vi "Image Processing.vi"(0 "Image In":T1, 7 "error in":errorcluster) -> (20 "Image Out":T1, 21 "Matches (Pattern Matching 1)":T2(array[cluster]) {"Bounding Box"."y" format="%.2f"; "Bounding Box"."x" format="%.2f"; "Position"."y" format="%.2f"; "Position"."x" format="%.2f"; "Score" format="%.2f"; "Scale" format="%.2f"; "Angle" format="%.2f"}, 27 "error out":errorcluster)   [LabVIEW 2018]
uses:
  <vilib>/vision/Image Controls.llb/IMAQ Image.ctl
  <vilib>/vision/Pattern Matching.llb/IMAQ Pattern Match Advanced Options.ctl
  <vilib>/vision/NI_Vision_Development_Module.lvlib
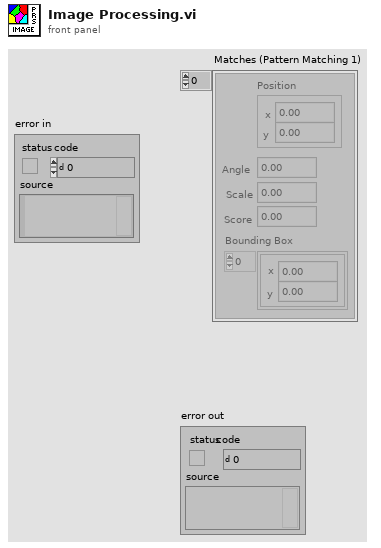
[diagram p1: front panel]
types:
  T1 = typedef "IMAQ Image.ctl" = refnum<image>
  T2 = cluster{"Position":cluster{"x":sgl, "y":sgl}, "Angle":sgl, "Scale":sgl, "Score":sgl, "Bounding Box":cluster{"x":sgl, "y":sgl}[]}[]
  T3 = typedef "IMAQ Pattern Match Advanced Options.ctl" = u16
  T4 = cluster{"Number of Matches Requested":i32, "Minimum Match Score":sgl, "Angle Ranges":cluster{"Start Angle":sgl, "End Angle":sgl}[]}
  T5 = cluster{"Global Rectangle":i32[], "Contours":cluster{"ID":enum32{"External", "Internal"}, "Type":u32, "Coordinates":i32[]}[]}
  T6 = cluster{"Global Rectangle":i32[], "Contours":cluster{"ID":enum32{"External", "Internal"}, "Type":u32, "Coordinates":i32[]}[]}[]
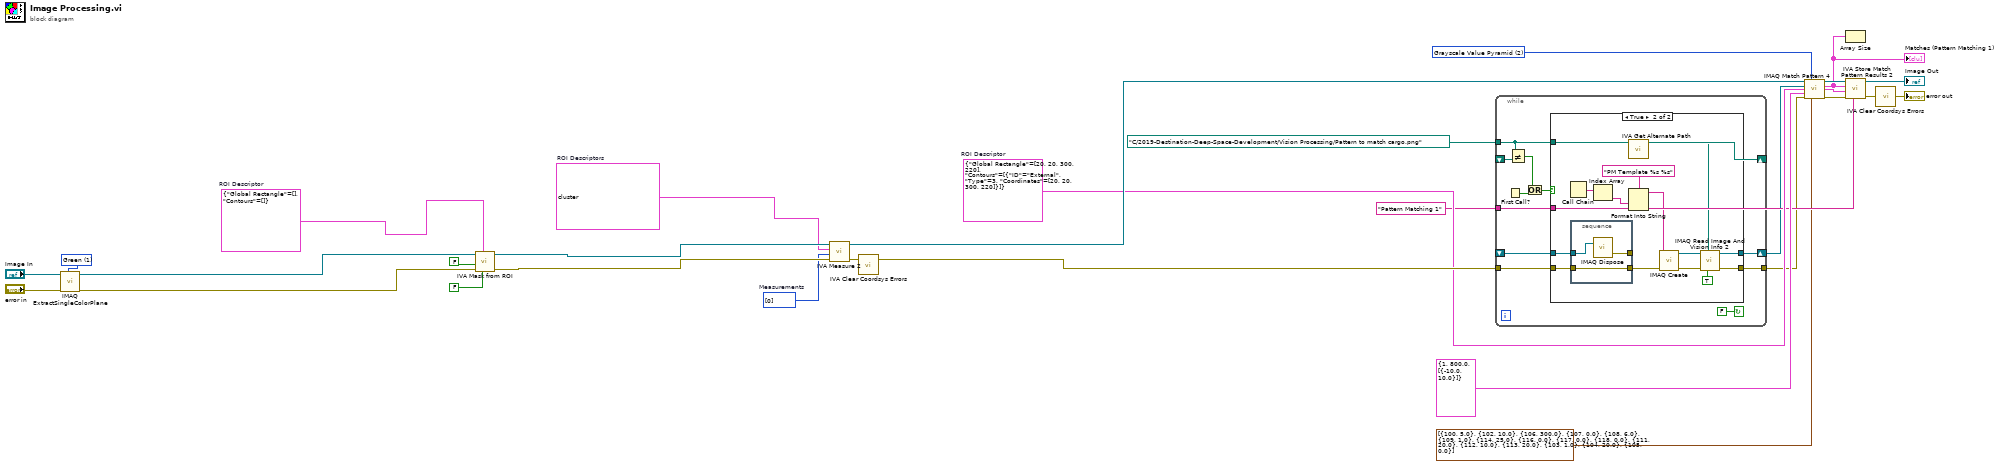
[diagram p0: block diagram]
diagram:
  w11 = 2 items=["All", "Low Discrepancy Sampling", "Grayscale Value Pyramid", "Gradients Pyramid"] ("Algorithm")
  w8 = "Pattern Matching 1" ("Step Name")
  w10 = T5 {"Global Rectangle"=[20, 20, 300, 220], "Contours"=[{"ID"=enum."External", "Type"=3, "Coordinates"=[20, 20, 300, 220]}]}  # ROI Descriptor
  w19 = i32[] [0]  # Measurements
  w20 = T6 [{"Global Rectangle"=[159, 103, 160, 104], "Contours"=[{"ID"=enum."External", "Type"=1, "Coordinates"=[159, 103]}]}]  # ROI Descriptors
  w26 = T5 {"Global Rectangle"=[], "Contours"=[]}  # ROI Descriptor
  w30 = 1 items=["Red", "Green", "Blue", "Hue", "Saturation", "Luminance", "Value", "Intensity"] ("Color Plane")
  n1 = call "IMAQ ExtractSingleColorPlane"("Color Plane"=w30, "error in (no error)"="error in", "Image Src"="Image In") -> ("error out"=w27:errorcluster, "Image Dst Out"=w24:T1)  [unwired: 1 in, 6 out]
  n2 = call <vilib>:"IVA Mask from ROI.vi"("Shrink"=FALSE, "ROI Descriptor"=w26, "error in (no error)"=w27, "Out / In"=FALSE, "Image Src"=w24) -> ("error out"=w22:errorcluster, "Image Out"=w21:T1)  [unwired: 5 out]
  n3 = call <vilib>:"IVA Measure 2.vi"("error in (no error)"=w22, "Measurements"=w19, "ROI Descriptors"=w20, "Image In"=w21) -> ("error out"=w18:errorcluster, "Image Out"=w15:T1)  [unwired: 1 in, 5 out]
  n4 = call <vilib>:"IVA Clear Coordsys Errors.vi"("error in (no error)"=w18) -> ("error out"=w17:errorcluster)  [unwired: 10 in]
  n5 = while {
    shift-right: [w41] -> w5
    shift-left: _ -> [w40]
    tunnel: [w38] -> w4
    tunnel: w17 -> [w37]
    tunnel: path "C:/2019-Destination-Deep-Space-Development/Vision Processing/Pattern to match cargo.png" ("Template File Path") -> [w34]
    tunnel: w8 -> [w36]
    shift-right: [w34] -> _
    shift-left: _ -> [w35]
    stop <- FALSE continue-if-true
    n6 = First Call?() -> (First Call?: T/F=w33:bool)
    n7 = Not Equal?(x=w34, y=w35) -> (x != y?=w32:bool)
    n8 = Or(x=w32, y=w33) -> (x .or. y?=w31:bool)
    n9 = case shown="True" w31 {
      tunnel: [w43 w48] -> w41
      tunnel: w40 -> [w43 w52]
      tunnel: [w42 w49] -> w38
      tunnel: w37 -> [w42 w51]
      tunnel: w34 -> [_ w53]
      tunnel: w36 -> [_ w54]
      frame False {
      }
      frame True {
        n10 = Call Chain() -> (call chain=w56:string[])
        n11 = stacked-sequence {
          tunnel: w52 -> [w61]
          tunnel: w51 -> [w60]
          tunnel: [w60] -> w45
          tunnel: [w59] -> _
          frame #0 {
            n12 = call "IMAQ Dispose"("Image"=w61) -> ("error out"=w59:errorcluster)  [unwired: 2 in, 3 out]
          }
        }
        n13 = Index Array(array=w56) -> (element=w55:string)  [unwired: 1 in]
        n14 = call <vilib>:"IVA Get Alternate Path.vi"("Path In"=w53) -> ("Path Out"=w50:path)  [unwired: 10 out]
        n15 = Format Into String(format string="PM Template %s %s" ("Image Name"), w55, w54) -> (resulting string=w58:string)  [unwired: 2 in, 1 out]
        n16 = call "IMAQ Create"("Image Name"=w58, "error in (no error)"=w45) -> ("New Image"=w47:T1, "error out"=w46:errorcluster)  [unwired: 2 in, 1 out]
        n17 = call "IMAQ Read Image And Vision Info 2"("Use File Path Image Type"=TRUE, "File Path"=w50, "error in (no error)"=w46, "Image"=w47) -> ("error out"=w49:errorcluster, "Image Out"=w48:T1)  [unwired: 5 in, 1 out]
      }
    }
  }
  n18 = call "IMAQ Match Pattern 4"("Image"=w15, "Algorithm"=w11, "Template Image"=w5, "ROI Descriptor"=w10, "Parameters"=T4 {"Number of Matches Requested"=1, "Minimum Match Score"=800.0, "Angle Ranges"=[{"Start Angle"=-10.0, "End Angle"=10.0}]}, "error in (no error)"=w4, "Advanced Options"=cluster{"Item":T3, "Value":dbl}[] [{"Item"=100, "Value"=5.0}, {"Item"=102, "Value"=10.0}, {"Item"=106, "Value"=300.0}, {"Item"=107, "Value"=0.0}, {"Item"=108, "Value"=6.0}, {"Item"=109, "Value"=1.0}, {"Item"=114, "Value"=25.0}, {"Item"=116, "Value"=0.0}, {"Item"=117, "Value"=0.0}, {"Item"=118, "Value"=0.0}, {"Item"=111, "Value"=20.0}, {"Item"=112, "Value"=10.0}, {"Item"=113, "Value"=20.0}, {"Item"=103, "Value"=1.0}, {"Item"=104, "Value"=20.0}, {"Item"=105, "Value"=0.0}]) -> ("Image (duplicate)"=w12:T1, "Matches (pixel)"=w7:T2, "Matches (real-world)"=w6:T2, "error out"=w13:errorcluster)  [unwired: 4 in, 1 out]
  "Matches (Pattern Matching 1)" <- w7
  n19 = Array Size(array=w7) -> ()  [unwired: 1 out]
  n20 = call <vilib>:"IVA Store Match Pattern Results 2.vi"("Step Name"=w8, "error in (no error)"=w13, "Matches (real-world)"=w6, "Matches (pixel)"=w7, "Image in"=w12) -> ("error out"=w3:errorcluster, "Image dup"=→"Image Out":T1)  [unwired: 1 in, 4 out]
  n21 = call <vilib>:"IVA Clear Coordsys Errors.vi"("error in (no error)"=w3) -> ("error out"=→"error out":errorcluster)  [unwired: 10 in]
